vi "Read TIO Count.vi"(4 "TL Calling Location":string, 6 "error In":errorcluster, 8 "taskID":u32, 9 "task IN":refnum<k21>) -> (0 "error out":errorcluster, 1 "timeout":bool, 2 "time (secs)":sgl format="%.8f", 3 "task out":refnum<k21>, 5 "count":u32)   [LabVIEW 2015]
doc: "DESCRIPTION:\nThis VI counts rising edges, using an NI-TIO based device (e.g.: 6602). The counter increments its event count everytime a pulse comes into its source input. The counters only increments between the rising edge of the aux line and the rising edge of the gate. The current value of the counter is read when the counter is finished or an error occurs. \n\n\n\nINSTRUCTIONS:\n1. Enter the device and counter you want use.\n2. Optional controls are located on the left side of the front panel. You will have to use your scroll bar to reach these. \n3. Connect your signals as described below in I/O CONNECTIONS.\n4. Run the VI.\n\n\nKEY PARAMETERS:\nCounter Group Config.vi: task type = two edge separation measurement\nCounter Source (NI-TIO).vi: Source Specification\nCounter Gate (NI-TIO).vi: Gate Specification\nCounter Aux Line (NI-TIO): Aux Line Specification\nCounter Get Attribute.vi: armed, TC Reached, count\nCounter Control.vi: Program, Reset\n\n\n\nI/O CONNECTIONS:\nConnect the start signal to the aux line input of the selected counter. Connect the stop signal to the gate input of the selected counter. \nIf you selected the Source Selection to be \"PFI line\", connect your event count base signal to the PFI line indicated by \"Source PFI line number used\". (If you selected \"Internal Timebase\", no source connection is necessary.)\n\nNOTE: For actual I/O pin numbers, please refer to your hardware user manual.\n\n\n\nDAQ VIs USED:\nCounter Group Config.vi\nCounter Source (NI-TIO).vi\nCounter Gate (NI-TIO).vi\nCounter Aux Line (NI-TIO)\nCounter Get Attribute.vi\nCounter Control.vi"
uses:
  <vilib>/Utility/error.llb/DialogType.ctl
  <vilib>/DAQmx/read.llb/DAQmx Read (Counter DBL 1Chan 1Samp).vi
  <vilib>/DAQmx/miscellaneous.llb/DAQmx Fill In Error Info.vi
panel:
  out "counter overflow?":bool
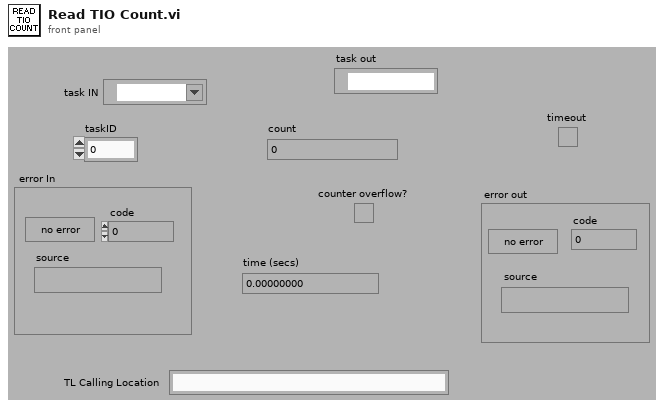
[diagram p1: front panel]
types:
  T1 = typedef "DialogType.ctl" = u16
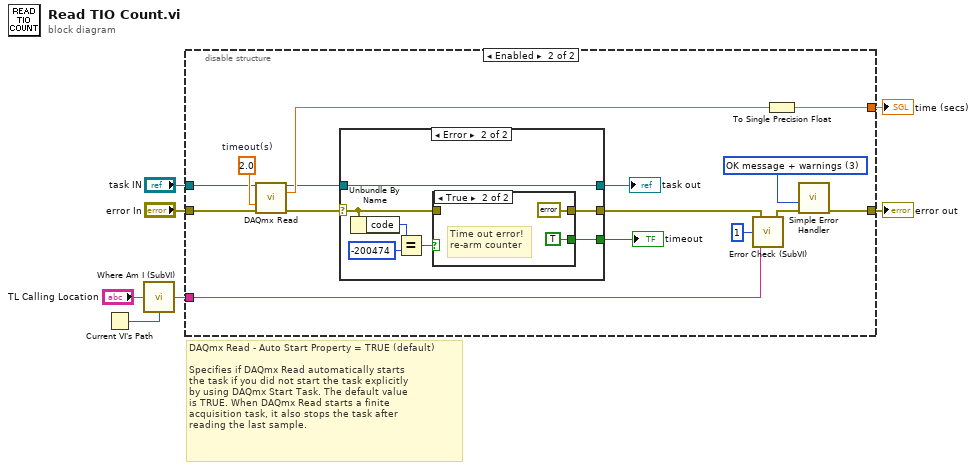
[diagram p0: block diagram]
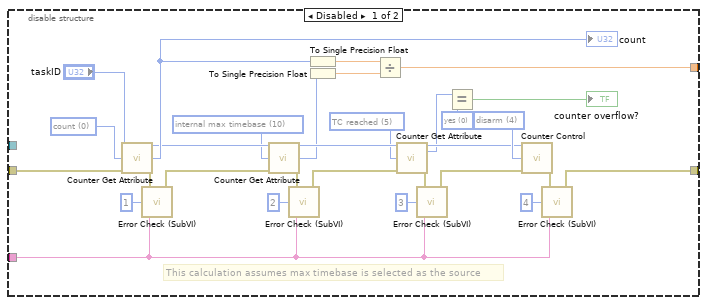
[diagram p2: hidden frame]
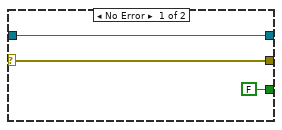
[diagram p3: hidden frame]
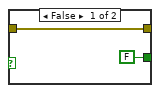
[diagram p4: hidden frame]
diagram:
  # "DAQmx Read - Auto Start Property = TRUE (default)\n\nSpecifies if DAQmx Read automatically starts \nthe task if you did not start the task explicitly \nby using DAQmx Start Task. The default value \nis TRUE. When DAQmx Read starts a finite \nacquisition task, it also stops the task after \nreading the last sample."
  n1 = Current VI's Path() -> (path=w4:path)
  n2 = call "Where Am I (SubVI).vi"("TL Calling Location"="TL Calling Location", "Call VI path"=w4) -> ("I'm here"=w2:string)
  n3 = disable-structure shown="Enabled" {
    disable-tunnel: "error In" -> [w32 w46]
    disable-tunnel: [w24 w47] -> w6
    disable-tunnel: [w9 w49] -> w5
    disable-tunnel: w2 -> [w8 w42]
    disable-tunnel: "task IN" -> [_ w48]
    frame Disabled {
      w27 = u32 0 items=["yes", "no", "high", "low"] ("attribute value type")
      w28 = u32 5 items=["count", "saved count", "count available", "available points", "armed", "TC reached", "done", "output state", "read mark", "write mark", "internal max timebase", "max prescale", "read mark high snapshot", "read mark low snapshot", "write mark high snapshot", "write mark low snapshot", "backlog high snapshot", "backlog low snapshot", "armed snapshot"] ("attribute ID")
      w29 = u32 10 items=["count", "saved count", "count available", "available points", "armed", "TC reached", "done", "output state", "read mark", "write mark", "internal max timebase", "max prescale", "read mark high snapshot", "read mark low snapshot", "write mark high snapshot", "write mark low snapshot", "backlog high snapshot", "backlog low snapshot", "armed snapshot"] ("attribute ID")
      w30 = u32 0 items=["count", "saved count", "count available", "available points", "armed", "TC reached", "done", "output state", "read mark", "write mark", "internal max timebase", "max prescale", "read mark high snapshot", "read mark low snapshot", "write mark high snapshot", "write mark low snapshot", "backlog high snapshot", "backlog low snapshot", "armed snapshot"] ("attribute ID")
      w37 = u32 4 items=["program", "reset", "arm", "prepare", "disarm", "count up", "count down", "switch cycle", "snapshot"] ("control code")
      # "This calculation assumes max timebase is selected as the source"
      n4 = call <vilib>:"Counter Get Attribute.vi"("task ID"="taskID", "attribute ID"=w30, "error in (no error)"=w32) -> ("task ID out"=w35:u32, "attribute value number"=w36:u32, "error out"=w19:errorcluster)  [unwired: 10 out]
      "count" <- w36
      n5 = call "Error Check (SubVI).vi"("calling VI"=w8, "tag #"=1 ("code locator tag #"), "error IN"=w19) -> ("error OUT"=w18:errorcluster)  [unwired: 2 out]
      n6 = call <vilib>:"Counter Get Attribute.vi"("task ID"=w35, "attribute ID"=w29, "error in (no error)"=w18) -> ("task ID out"=w34:u32, "attribute value number"=w23:u32, "error out"=w13:errorcluster)  [unwired: 10 out]
      n7 = call "Error Check (SubVI).vi"("calling VI"=w8, "tag #"=2 ("code locator tag #"), "error IN"=w13) -> ("error OUT"=w12:errorcluster)  [unwired: 2 out]
      n8 = To Single Precision Float(number=w36) -> (single precision float=w22:sgl)
      n9 = To Single Precision Float(number=w23) -> (single precision float=w21:sgl)
      n10 = Divide(x=w22, y=w21) -> (x/y=w24:sgl)
      n11 = call <vilib>:"Counter Get Attribute.vi"("task ID"=w34, "attribute ID"=w28, "error in (no error)"=w12) -> ("task ID out"=w33:u32, "attribute value type"=w26:u32, "error out"=w11:errorcluster)  [unwired: 10 out]
      n12 = call "Error Check (SubVI).vi"("calling VI"=w8, "tag #"=3 ("code locator tag #"), "error IN"=w11) -> ("error OUT"=w10:errorcluster)  [unwired: 2 out]
      n13 = Equal?(x=w26, y=w27) -> (x = y?=→"counter overflow?":bool)
      n14 = call <vilib>:"Counter Control.vi"("task ID"=w33, "control code"=w37, "error in (no error)"=w10) -> ("error out"=w14:errorcluster)  [unwired: 12 out]
      n15 = call "Error Check (SubVI).vi"("calling VI"=w8, "tag #"=4 ("code locator tag #"), "error IN"=w14) -> ("error OUT"=w9:errorcluster)  [unwired: 2 out]
    }
    frame Enabled {
      w51 = T1 3 items=["no dialog", "OK message", "continue or stop message", "OK message + warnings", "continue/stop + warnings"] ("type of dialog (OK msg:1)")
      w52 = 2.0  # timeout(s)
      n16 = call-poly <vilib>:"DAQmx Read.vi"("task/channels in"=w48, "timeout"=w52, "error in"=w46) -> ("task out"=w45:refnum<k21>, "data"=w50:dbl, "error out"=w44:errorcluster)  [unwired: 10 in]
      n17 = case shown="Error" w44 {
        selector: w44 -> [w54 w58]
        tunnel: w45 -> [w55 w62]
        tunnel: [w55 w62] -> w40
        tunnel: [w54 w57] -> w41
        tunnel: [FALSE ("timeout") w56] -> w38
        frame No Error {
        }
        frame Error {
          n18 = Unbundle By Name(w58) -> ("code"=w61:i32)
          n19 = Equal?(x=w61, y=-200474) -> (x = y?=w59:bool)
          n20 = case shown="True" w59 {
            tunnel: w58 -> [w64 _]
            tunnel: [w64 errorcluster {"status"=FALSE, "code"=0, "source"=""} ("error IO")] -> w57
            tunnel: [FALSE ("timeout") TRUE ("timeout")] -> w56
            frame False {
            }
            frame True {
              # "Time out error!\nre-arm counter"
            }
          }
        }
      }
      "task out" <- w40
      "timeout" <- w38
      n21 = call "Error Check (SubVI).vi"("calling VI"=w42, "tag #"=1 ("code locator tag #"), "error IN"=w41) -> ("error OUT"=w39:errorcluster)  [unwired: 2 out]
      n22 = To Single Precision Float(number=w50) -> (single precision float=w47:sgl)
      n23 = call <vilib>:"Simple Error Handler.vi"("type of dialog (OK msg:1)"=w51, "error in (no error)"=w39) -> ("error out"=w49:errorcluster)  [unwired: 3 in, 4 out]
    }
  }
  "time (secs)" <- w6
  "error out" <- w5
